vi "i2c tester.vi"() -> ()   [LabVIEW 2014]
uses:
  Type Defs/VL6180X DEFS.ctl
  Type Defs/VL6180 Resource.ctl
  <vilib>/MakerHub/LINX/Private/Type Defs/LINX Ref.ctl
  <vilib>/MakerHub/LINX/Private/Type Defs/Platform.ctl
  <vilib>/MakerHub/LINX/Private/Type Defs/Interface.ctl
  <vilib>/MakerHub/LINX/Private/Device/Type Defs/LINX Device Config.ctl
  <vilib>/MakerHub/LINX/Private/Device/Type Defs/TCP Config.ctl
  <vilib>/MakerHub/LINX/Private/Device/Type Defs/Channels.ctl
  <vilib>/MakerHub/LINX/Public/Utilities/Open Local.vi
  <vilib>/MakerHub/LINX/LMH-LINX.lvlib
  <vilib>/MakerHub/LINX/Public/Peripherals/Digital/Digital Write 1 Chan.vi
  <vilib>/MakerHub/LINX/Private/Device/Device.lvlib
panel:
  out "Data out":u8 format="%02x"
  in  "I2C Slave Address (0) 2":u8=41 format="%x"
  in  "I2C Channel 2":u8=1
  in  "VL6180 PWR Channel":u8=35
  in  "Power VL6180":bool
  in  "Input":u16=22 format="%04x"
  in  "stop":bool
  out "Data":u16 format="%04x"
  in  "I2C Slave Address (0)":u8=41 format="%x"
  in  "I2C Channel":u8=1
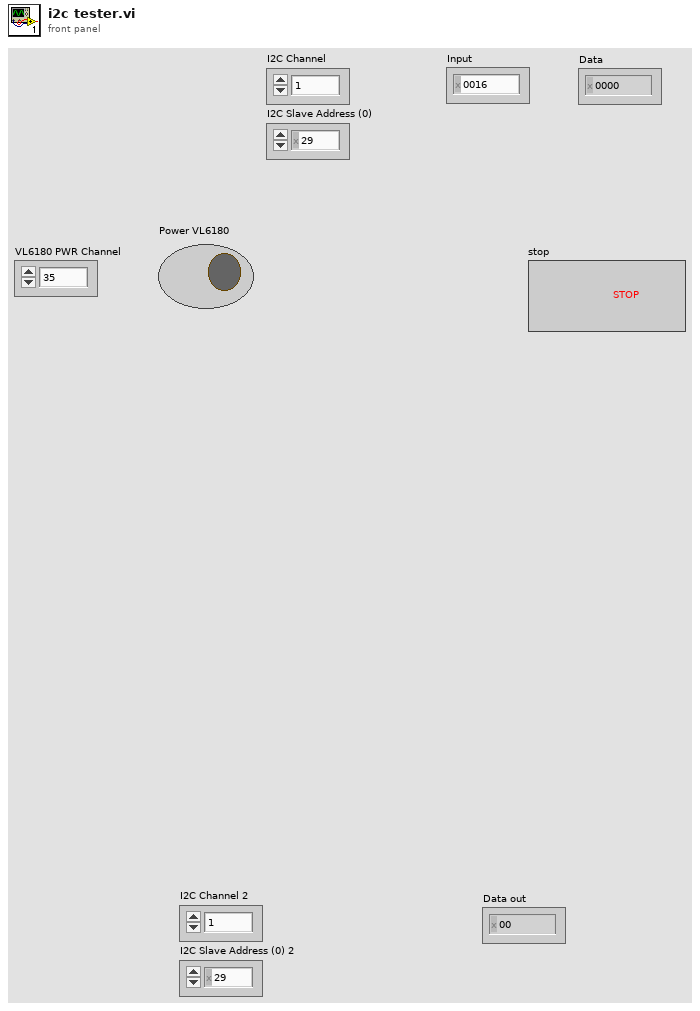
[diagram p1: front panel]
types:
  T1 = typedef "VL6180 Resource.ctl" = cluster{"LINX Resource":T2, "I2C Channel":u8, "I2C Slave Address":u8}
  T2 = typedef "LMH-LINX.lvlib/LINX Ref.ctl" = cluster{"IO":T3, "Interface":T4, "LINX Device Config":T5}
  T3 = typedef "LMH-LINX.lvlib/Platform.ctl" = enum16{"Remote", "Local"}
  T4 = typedef "LMH-LINX.lvlib/Interface.ctl" = enum16{"Serial", "TCP"}
  T5 = typedef "LMH-LINX.lvlib/Device.lvlib/LINX Device Config.ctl" = cluster{"Interface":T4, "COM Port":refnum<visa-resource-name>, "TCP Configuration":T6, "Device Family":u8, "Device ID":u8, "Device Name":string, "TCP Ref":refnum<k5>, "Channels":T7}
  T6 = typedef "LMH-LINX.lvlib/Device.lvlib/TCP Config.ctl" = cluster{"IP Address":string, "Port":u16}
  T7 = typedef "LMH-LINX.lvlib/Channels.ctl" = cluster{"DI":u8[], "DO":u8[], "AI":u8[], "AO":u8[], "PWM":u8[], "QE":u8[], "UART":u8[], "I2C 2":u8[], "SPI":u8[], "CAN":u8[], "Servo":u8[], "AI Ref (V)":dbl, "AI Resolution (Bits)":u8, "AO Ref (V)":dbl, "AO Resolution (Bits)":u8}
  T8 = typedef "VL6180X DEFS.ctl" = u16
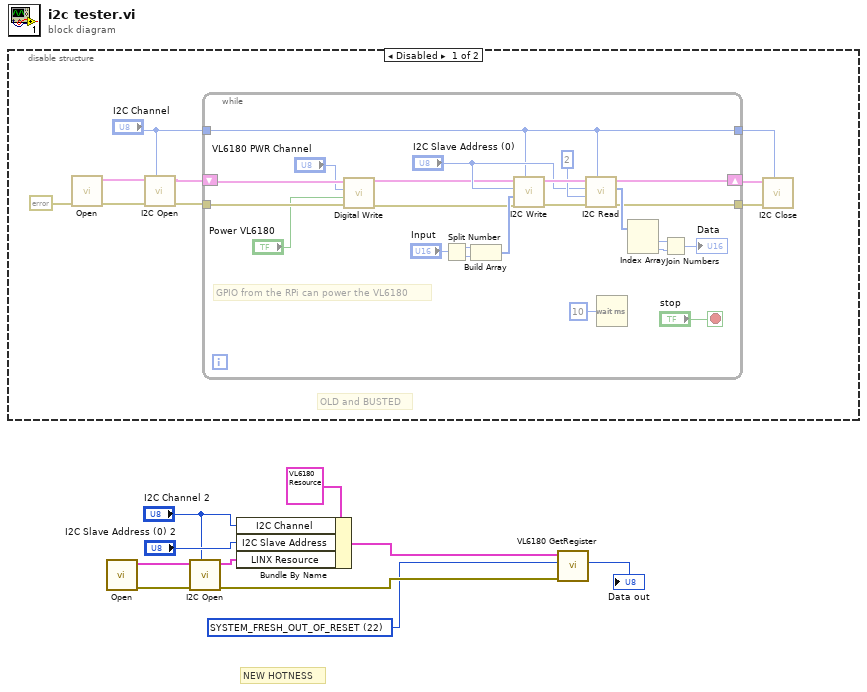
[diagram p0: block diagram]
diagram:
  w2 = T8 22 items=["IDENTIFICATION_MODEL_ID"=0, "IDENTIFICATION_MODEL_REV_MAJOR"=1, "IDENTIFICATION_MODEL_REV_MINOR"=2, "IDENTIFICATION_MODULE_REV_MAJOR"=3, "IDENTIFICATION_MODULE_REV_MINOR"=4, "IDENTIFICATION_DATE"=6, "IDENTIFICATION_TIME"=8, "SYSTEM_MODE_GPIO0"=16, "SYSTEM_MODE_GPIO1"=17, "SYSTEM_HISTORY_CTRL"=18, "SYSTEM_INTERRUPT_CONFIG_GPIO"=20, "SYSTEM_INTERRUPT_CLEAR"=21, "SYSTEM_FRESH_OUT_OF_RESET"=22, "SYSTEM_GROUPED_PARAMETER_HOLD"=23, "SYSRANGE_START"=24, "SYSRANGE_THRESH_HIGH"=25, "SYSRANGE_THRESH_LOW"=26, "SYSRANGE_INTERMEASUREMENT_PERIOD"=27, "SYSRANGE_MAX_CONVERGENCE_TIME"=28, "SYSRANGE_CROSSTALK_COMPENSATION_RATE"=30, "SYSRANGE_CROSSTALK_VALID_HEIGHT"=33, "SYSRANGE_EARLY_CONVERGENCE_ESTIMATE"=34, "SYSRANGE_PART_TO_PART_RANGE_OFFSET"=36, "SYSRANGE_RANGE_IGNORE_VALID_HEIGHT"=37, "SYSRANGE_RANGE_IGNORE_THRESHOLD"=38, "SYSRANGE_MAX_AMBIENT_LEVEL_MULT"=44, "SYSRANGE_RANGE_CHECK_ENABLES"=45, "SYSRANGE_VHV_RECALIBRATE"=46, "SYSRANGE_VHV_REPEAT_RATE"=49, "SYSALS_START"=56, "SYSALS_THRESH_HIGH"=58, "SYSALS_THRESH_LOW"=60, "SYSALS_INTERMEASUREMENT_PERIOD"=62, "SYSALS_ANALOGUE_GAIN"=63, "SYSALS_INTEGRATION_PERIOD"=64, "RESULT_RANGE_STATUS"=77, "RESULT_ALS_STATUS"=78, "RESULT_INTERRUPT_STATUS_GPIO"=79, "RESULT_ALS_VAL"=80, "RESULT_HISTORY_BUFFER"=82, "RESULT_RANGE_VAL"=98, "RESULT_RANGE_RAW"=100, "RESULT_RANGE_RETURN_RATE"=102, "RESULT_RANGE_REFERENCE_RATE"=104, "RESULT_RANGE_RETURN_SIGNAL_COUNT"=108, "RESULT_RANGE_REFERENCE_SIGNAL_COUNT"=112, "RESULT_RANGE_RETURN_AMB_COUNT"=116, "RESULT_RANGE_REFERENCE_AMB_COUNT"=120, "RESULT_RANGE_RETURN_CONV_TIME"=124, "RESULT_RANGE_REFERENCE_CONV_TIME"=128, "READOUT_AVERAGING_SAMPLE_PERIOD"=266, "FIRMWARE_BOOTUP"=281, "FIRMWARE_RESULT_SCALER"=288, "I2C_SLAVE_DEVICE_ADDRESS"=530, "INTERLEAVED_MODE_ENABLE"=675] ("VL6180X Constants")
  # "NEW HOTNESS"
  n1 = disable-structure shown="Disabled" {
    frame Disabled {
      # "OLD and BUSTED"
      n2 = call-poly <vilib>:"Open.vi"("Error In"=errorcluster {"status"=FALSE, "code"=0, "source"=""}) -> ("Error Out"=w18:errorcluster, "LINX Resource"=w19:T2)  [unwired: 8 in, 1 out]
      n3 = call <vilib>:"I2C Open.vi"("I2C Channel (0)"="I2C Channel", "Error In"=w18, "LINX Resource"=w19) -> ("Error Out"=w16:errorcluster, "LINX Resource"=w17:T2)  [unwired: 7 in]
      n4 = while {
        shift-right: [w33] -> w15
        shift-left: w17 -> [w23]
        tunnel: [w27] -> w13
        tunnel: "I2C Channel" -> [w27]
        tunnel: w16 -> [w26]
        tunnel: [w34] -> w14
        stop <- "stop" stop-if-true
        # "GPIO from the RPi can power the VL6180"
        n5 = call-poly <vilib>:"Digital Write.vi"("Error In"=w26, "Output Value"="Power VL6180", "DO Channel"="VL6180 PWR Channel", "LINX Resource"=w23) -> ("Error Out"=w25:errorcluster, "LINX Resource"=w24:T2)  [unwired: 6 in]
        n6 = Split Number(x="Input") -> (hi(x)=w30:u8, lo(x)=w29:u8)
        n7 = Build Array(w30, w29) -> (w28:u8[])
        n8 = call <vilib>:"I2C Write.vi"("I2C Channel"=w27, "Error In"=w25, "Data"=w28, "I2C Slave Address (0)"="I2C Slave Address (0)", "LINX Resource"=w24) -> ("Error Out"=w41:errorcluster, "LINX Resource"=w42:T2)  [unwired: 5 in]
        n9 = call <vilib>:"I2C Read.vi"("I2C Channel"=w27, "Error In"=w41, "Bytes To Read"=u8 2, "I2C Slave Address (0)"="I2C Slave Address (0)", "LINX Resource"=w42) -> ("Error Out"=w34:errorcluster, "Data"=w37:u8[], "LINX Resource"=w33:T2)  [unwired: 4 in]
        n10 = Wait (ms)(milliseconds to wait=u32 10) -> ()  [unwired: 1 out]
        n11 = Index Array(array=w37) -> (element #1=w38:u8, element #2=w36:u8)  [unwired: 2 in]
        n12 = Join Numbers(hi=w38, lo=w36) -> ((hi.lo)=→"Data":u16)
      }
      n13 = call <vilib>:"I2C Close.vi"("I2C Channel (0)"=w13, "Error In"=w14, "LINX Resource"=w15) -> ()  [unwired: 7 in, 2 out]
    }
    frame Enabled {
    }
  }
  n14 = call-poly <vilib>:"Open.vi"() -> ("Error Out"=w4:errorcluster, "LINX Resource"=w5:T2)  [unwired: 9 in, 1 out]
  n15 = call <vilib>:"I2C Open.vi"("I2C Channel (0)"="I2C Channel 2", "Error In"=w4, "LINX Resource"=w5) -> ("Error Out"=w10:errorcluster, "LINX Resource"=w8:T2)  [unwired: 7 in]
  n16 = Bundle By Name(cluster=T1 {"LINX Resource"={"IO"=enum."Remote", "Interface"=enum."Serial", "LINX Device Config"={"Interface"=enum."Serial", "COM Port"="", "TCP Configuration"={"IP Address"="", "Port"=0}, "Device Family"=0, "Device ID"=0, "Device Name"="", "TCP Ref"=refnum, "Channels"={"DI"=[], "DO"=[], "AI"=[], "AO"=[], "PWM"=[], "QE"=[], "UART"=[], "I2C 2"=[], "SPI"=[], "CAN"=[], "Servo"=[], "AI Ref (V)"=0.0, "AI Resolution (Bits)"=0, "AO Ref (V)"=0.0, "AO Resolution (Bits)"=0}}}, "I2C Channel"=0, "I2C Slave Address"=0} ("VL6180 Resource"), "I2C Channel"="I2C Channel 2", "I2C Slave Address"="I2C Slave Address (0) 2", "LINX Resource"=w8) -> (w7:T1)
  n17 = call "VL6180 GetRegister.vi"("error in"=w10, "VL6180X Constants"=w2, "VL6180 Resource"=w7) -> ("Data out"=→"Data out":u8)  [unwired: 6 in, 2 out]
